vi "Script Add Constant VI.vi"(4 "Project Ref":refnum<vi>, 6 "App Ref":refnum<vi>, 7 "Constant VI Name":string="TESTING.vi", 8 "error in":errorcluster, 9 "Constant VI Args":refnum<vi>, 10 "DQMH Lib Ref":refnum<vi>) -> (0 "error out":errorcluster, 3 "VI out":refnum<class "VI.lvclass">)   [LabVIEW 2019, in "Panther Dashboard.lvlib"]
uses:
  Panther Dashboard.lvlib
  Class/VI/VI.lvclass
  Class/LabVIEWItem/Item Type--enum.ctl
  Class/LabVIEWItem/LabVIEWItem.lvclass
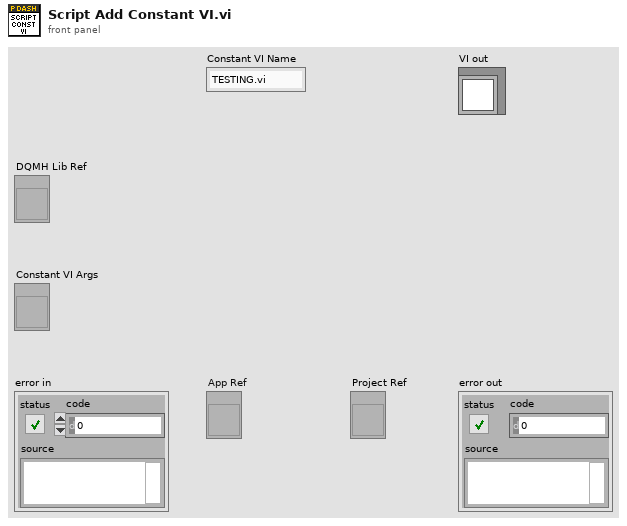
[diagram p1: front panel]
types:
  T1 = typedef "Panther Dashboard.lvlib/LabVIEWItem.lvclass/Item Type--enum.ctl" = enum16{"Requests", "Broadcasts", "Request and Wait for Reply", "Round Trip", "Public API VIs", "» Constant VIs", "» Error VIs", "Module", "Project"}
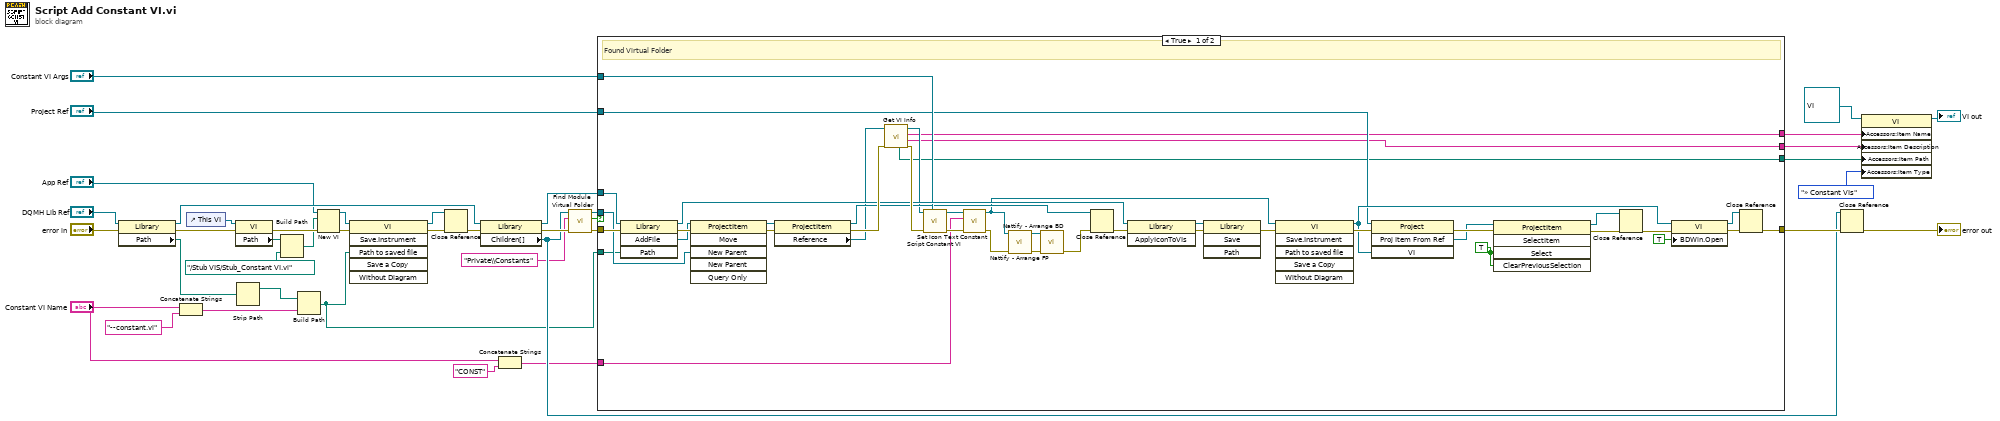
[diagram p0: block diagram]
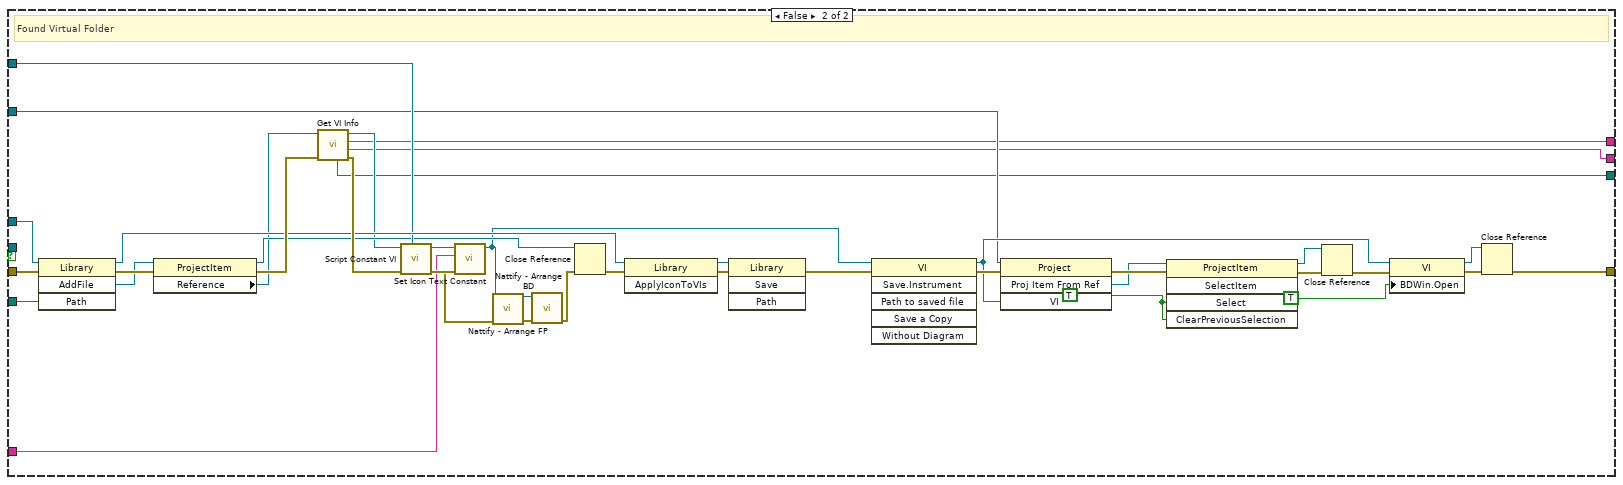
[diagram p2: hidden frame]
diagram:
  n1 = property class="Library"(reference="DQMH Lib Ref", error in="error in") -> (reference out=w29:refnum<vi>, error out=w37:errorcluster, "Path"=w18:path)
  n2 = Concatenate Strings("Constant VI Name", "--constant.vi" ("input 1")) -> (w17:string)
  n3 = control-ref of="This VI"() -> (w16:refnum<vi>)
  n4 = property class="VI"(reference=w16, error in=w37) -> (error out=w31:errorcluster, "Path"=w15:path)  [unwired: 1 out]
  n5 = Strip Path(path=w18) -> (stripped path=w20:path)  [unwired: 1 out]
  n6 = Build Path(base path=w15, name or relative path=path "../Stub VIS/Stub_Constant VI.vi") -> (appended path=w14:path)
  n7 = Build Path(base path=w20, name or relative path=w17) -> (appended path=w19:path)
  n8 = New VI(8:w31, 10:w14, 11:"App Ref") -> (0:w34:errorcluster, 3:w22:refnum<vi>)  [unwired: 4 in]
  n9 = invoke class="VI" method="Save.Instrument"(reference=w22, error in=w34, "Path to saved file"=w19) -> (reference out=w12:refnum<vi>, error out=w32:errorcluster)  [unwired: 3 in, 4 out]
  n10 = Close Reference(reference=w12, error in (no error)=w32) -> (error out=w33:errorcluster)
  n11 = property class="Library"(reference=w29, error in=w33) -> (reference out=w30:refnum<vi>, error out=w39:errorcluster, "Children[]"=w26:refnum<vi>[])
  n12 = Concatenate Strings("Constant VI Name", "CONST" ("string")) -> (w8:string)
  n13 = call "Find Module Virtual Folder.vi"("error in"=w39, "Virtual Folder"="Private\\Constants", "Children[]"=w26) -> ("error out"=w38:errorcluster, "Found?"=w27:bool, "ProjectItem out"=w28:refnum<vi>)  [unwired: 6 in]
  n14 = case shown="True" w27 {
    tunnel: [w72 w113] -> w40
    tunnel: w30 -> [w65 w106]
    tunnel: w38 -> [w83 w123]
    tunnel: w28 -> [w63 _]
    tunnel: "Constant VI Args" -> [w59 w101]
    tunnel: w19 -> [w60 w102]
    tunnel: w8 -> [w51 w94]
    tunnel: "Project Ref" -> [w46 w90]
    tunnel: [w43 w86] -> w3
    tunnel: [w42 w85] -> w2
    tunnel: [w41 w84] -> w1
    frame True {
      w49 = TRUE ("Select")
      # "Found Virtual Folder"
      n15 = invoke class="Library" method="AddFile"(reference=w65, error in=w83, "Path"=w60) -> (reference out=w62:refnum<vi>, error out=w82:errorcluster, "AddFile"=w64:refnum<vi>)  [unwired: 1 in, 1 out]
      n16 = invoke class="ProjectItem" method="Move"(reference=w64, error in=w82, "New Parent"=w63) -> (reference out=w57:refnum<vi>, error out=w79:errorcluster)  [unwired: 3 in, 4 out]
      n17 = property class="ProjectItem"(reference=w57, error in=w79) -> (reference out=w56:refnum<vi>, error out=w67:errorcluster, "Reference"=w45:refnum<vi>)
      n18 = call "Get VI Info.vi"("error in"=w67, "VI in"=w45) -> ("error out"=w66:errorcluster, "VI Description"=w42:string, "Plain Name"=w43:string, "VI out"=w44:refnum<vi>, "VI Path"=w41:path)  [unwired: 4 in, 1 out]
      n19 = call "Script Constant VI.vi"("Custom Argument Window"=w59, "error in"=w66, "VI Reference"=w44) -> ("error out"=w78:errorcluster, "VI reference"=w58:refnum<vi>)  [unwired: 7 in]
      n20 = call "Set Icon Text Constant.vi"("error in"=w78, "Text"=w51, "VI in"=w58) -> ("error out"=w76:errorcluster, "VI out"=w54:refnum<vi>)  [unwired: 7 in]
      n21 = call "Nattify - Arrange FP.vi"("VI in"=w54, "error in"=w76) -> ("VI out"=w55:refnum<vi>, "error out"=w77:errorcluster)  [unwired: 12 in]
      n22 = call "Nattify - Arrange BD.vi"("VI in"=w55, "error in"=w77) -> ("error out"=w74:errorcluster)  [unwired: 13 in]
      n23 = Close Reference(reference=w56, error in (no error)=w74) -> (error out=w80:errorcluster)
      n24 = invoke class="Library" method="ApplyIconToVIs"(reference=w62, error in=w80) -> (reference out=w61:refnum<vi>, error out=w81:errorcluster)  [unwired: 1 in, 1 out]
      n25 = invoke class="Library" method="Save"(reference=w61, error in=w81) -> (error out=w73:errorcluster)  [unwired: 2 in, 3 out]
      n26 = invoke class="VI" method="Save.Instrument"(reference=w54, error in=w73) -> (reference out=w48:refnum<vi>, error out=w70:errorcluster)  [unwired: 4 in, 4 out]
      n27 = invoke class="Project" method="Proj Item From Ref"(reference=w46, error in=w70, "VI"=w48) -> (error out=w71:errorcluster, "ProjItemFromRef"=w50:refnum<vi>)  [unwired: 1 in, 2 out]
      n28 = invoke class="ProjectItem" method="SelectItem"(reference=w50, error in=w71, "Select"=w49, "ClearPreviousSelection"=w49) -> (reference out=w47:refnum<vi>, error out=w69:errorcluster)  [unwired: 1 in, 3 out]
      n29 = Close Reference(reference=w47, error in (no error)=w69) -> (error out=w68:errorcluster)
      n30 = property class="VI"(reference=w48, error in=w68, "BDWin.Open"=TRUE ("Block Diagram Window:Open")) -> (reference out=w52:refnum<vi>, error out=w75:errorcluster)
      n31 = Close Reference(reference=w52, error in (no error)=w75) -> (error out=w72:errorcluster)
    }
    frame False {
      w92 = TRUE ("Select")
      # "Found Virtual Folder"
      n32 = invoke class="Library" method="AddFile"(reference=w106, error in=w123, "Path"=w102) -> (reference out=w104:refnum<vi>, error out=w112:errorcluster, "AddFile"=w105:refnum<vi>)  [unwired: 1 in, 1 out]
      n33 = property class="ProjectItem"(reference=w105, error in=w112) -> (reference out=w99:refnum<vi>, error out=w119:errorcluster, "Reference"=w88:refnum<vi>)
      n34 = call "Get VI Info.vi"("error in"=w119, "VI in"=w88) -> ("error out"=w107:errorcluster, "VI Description"=w85:string, "Plain Name"=w86:string, "VI out"=w87:refnum<vi>, "VI Path"=w84:path)  [unwired: 4 in, 1 out]
      n35 = call "Script Constant VI.vi"("Custom Argument Window"=w101, "error in"=w107, "VI Reference"=w87) -> ("error out"=w120:errorcluster, "VI reference"=w100:refnum<vi>)  [unwired: 7 in]
      n36 = call "Set Icon Text Constant.vi"("error in"=w120, "Text"=w94, "VI in"=w100) -> ("error out"=w117:errorcluster, "VI out"=w97:refnum<vi>)  [unwired: 7 in]
      n37 = call "Nattify - Arrange FP.vi"("VI in"=w97, "error in"=w117) -> ("VI out"=w98:refnum<vi>, "error out"=w118:errorcluster)  [unwired: 12 in]
      n38 = call "Nattify - Arrange BD.vi"("VI in"=w98, "error in"=w118) -> ("error out"=w115:errorcluster)  [unwired: 13 in]
      n39 = Close Reference(reference=w99, error in (no error)=w115) -> (error out=w121:errorcluster)
      n40 = invoke class="Library" method="ApplyIconToVIs"(reference=w104, error in=w121) -> (reference out=w103:refnum<vi>, error out=w122:errorcluster)  [unwired: 1 in, 1 out]
      n41 = invoke class="Library" method="Save"(reference=w103, error in=w122) -> (error out=w114:errorcluster)  [unwired: 2 in, 3 out]
      n42 = invoke class="VI" method="Save.Instrument"(reference=w97, error in=w114) -> (reference out=w91:refnum<vi>, error out=w110:errorcluster)  [unwired: 4 in, 4 out]
      n43 = invoke class="Project" method="Proj Item From Ref"(reference=w90, error in=w110, "VI"=w91) -> (error out=w111:errorcluster, "ProjItemFromRef"=w93:refnum<vi>)  [unwired: 1 in, 2 out]
      n44 = invoke class="ProjectItem" method="SelectItem"(reference=w93, error in=w111, "Select"=w92, "ClearPreviousSelection"=w92) -> (reference out=w89:refnum<vi>, error out=w109:errorcluster)  [unwired: 1 in, 3 out]
      n45 = Close Reference(reference=w89, error in (no error)=w109) -> (error out=w108:errorcluster)
      n46 = property class="VI"(reference=w91, error in=w108, "BDWin.Open"=TRUE ("Block Diagram Window:Open")) -> (reference out=w95:refnum<vi>, error out=w116:errorcluster)
      n47 = Close Reference(reference=w95, error in (no error)=w116) -> (error out=w113:errorcluster)
    }
  }
  n48 = Close Reference(reference=w26, error in (no error)=w40) -> (error out=→"error out":errorcluster)
  n49 = property class="VI"(reference=refnum<class "VI.lvclass"> refnum ("VI"), "Accessors:Item Name"=w3, "Accessors:Item Description"=w2, "Accessors:Item Path"=w1, "Accessors:Item Type"=Item_Type--enum."» Constant VIs" ("Item Type")) -> (reference out=→"VI out":refnum<class "VI.lvclass">)  [unwired: 1 in, 1 out]
